vi "SngJntArmSim_GetCurrentDraw.vi"(11 "SingleJointArmSim":T1 {"GearBox"."Jr_KgM2" format="%13.5p"; "GearBox"."L_H" format="%13.5p"; "GearBox"."Kt_NMPerAmp" format="%13.5p"; "GearBox"."KvINV_RadPerSecPerVolt" format="%13.5p"; "GearBox"."R_Ohms" format="%13.5p"; "GearBox"."FreeSpeed_RadPerSec" format="%13.5p"; "GearBox"."FreeCurrent_Amps" format="%13.5p"; "GearBox"."StallCurrent_Amps" format="%13.5p"; "GearBox"."StallTorque_NM" format="%13.5p"; "GearBox"."nominalVoltage_Volts" format="%13.5p"}) -> (3 "Current_Amps":dbl)   [LabVIEW 2019, in "Trajectory_Library.lvlib"]
doc: "Returns the arm current draw.\n \nInputs:\n - SingleJointArmSim -- updated system data cluster\n\nOutputs:\n - Current_Amps -- The aram current draw. (Amps)"
uses:
  Trajectory_Library.lvlib
  SINGLE_JOINT_ARM_SIM.ctl
  LINEAR_SYSTEM_SIM.ctl
  LINEAR_SYSTEM.ctl
  <vilib>/Analysis/Matrix/Datatypes/RealMatrix.ctl
  DCMOTOR.CTL
  <vilib>/Analysis/Matrix/NI_Matrix.lvlib
panel:
  # "<States, 1>"
  # "<Outputs, 1>"
  # "<Inputs, 1>"
  # "<Outputs, 1>"
  # "<States,States>"
  # "<States,Inputs>"
  # "<Outputs,States>"
  # "<Outputs,Inputs>"
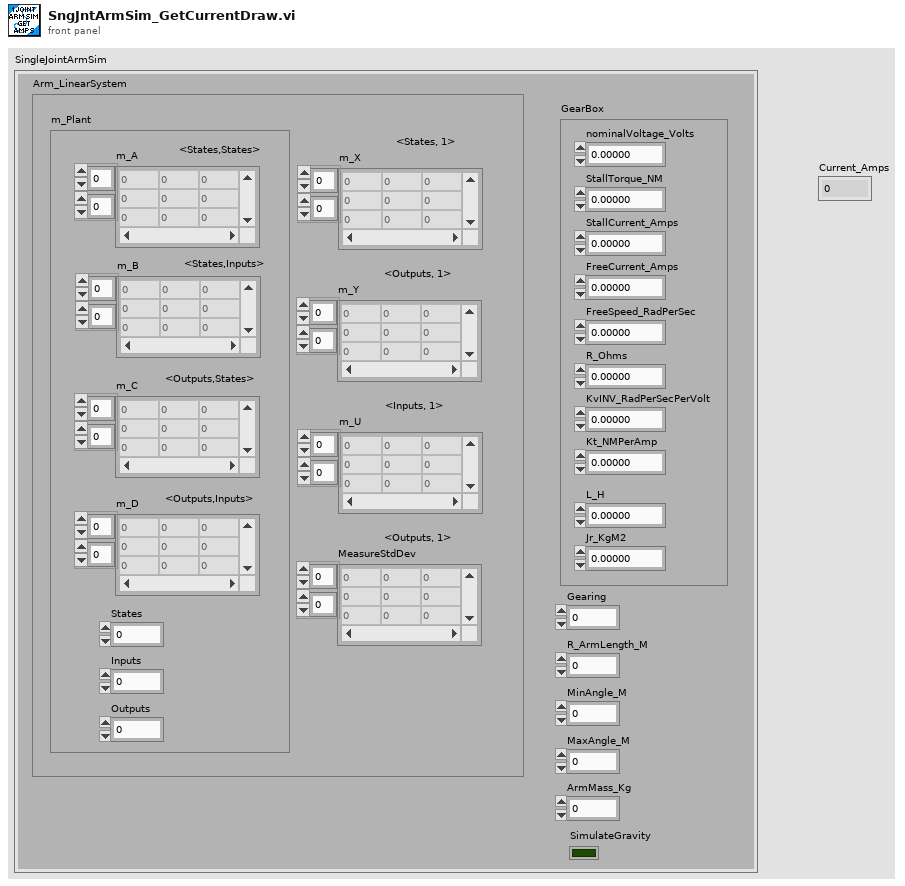
[diagram p1: front panel]
types:
  T1 = typedef "Trajectory_Library.lvlib/SINGLE_JOINT_ARM_SIM.ctl" = cluster{"Arm_LinearSystem":T2, "GearBox":T5, "Gearing":dbl, "R_ArmLength_M":dbl, "MinAngle_M":dbl, "MaxAngle_M":dbl, "ArmMass_Kg":dbl, "SimulateGravity":bool}
  T2 = typedef "Trajectory_Library.lvlib/LINEAR_SYSTEM_SIM.ctl" = cluster{"m_Plant":T3, "m_X":T4, "m_Y":T4, "m_U":T4, "MeasureStdDev":T4}
  T3 = typedef "Trajectory_Library.lvlib/LINEAR_SYSTEM.ctl" = cluster{"m_A":T4, "m_B":T4, "m_C":T4, "m_D":T4, "States":i32, "Inputs":i32, "Outputs":i32}
  T4 = typedef "NI_Matrix.lvlib/RealMatrix.ctl" = dbl[][]
  T5 = typedef "Trajectory_Library.lvlib/DCMOTOR.CTL" = cluster{"nominalVoltage_Volts":dbl, "StallTorque_NM":dbl, "StallCurrent_Amps":dbl, "FreeCurrent_Amps":dbl, "FreeSpeed_RadPerSec":dbl, "R_Ohms":dbl, "KvINV_RadPerSecPerVolt":dbl, "Kt_NMPerAmp":dbl, "L_H":dbl, "Jr_KgM2":dbl}
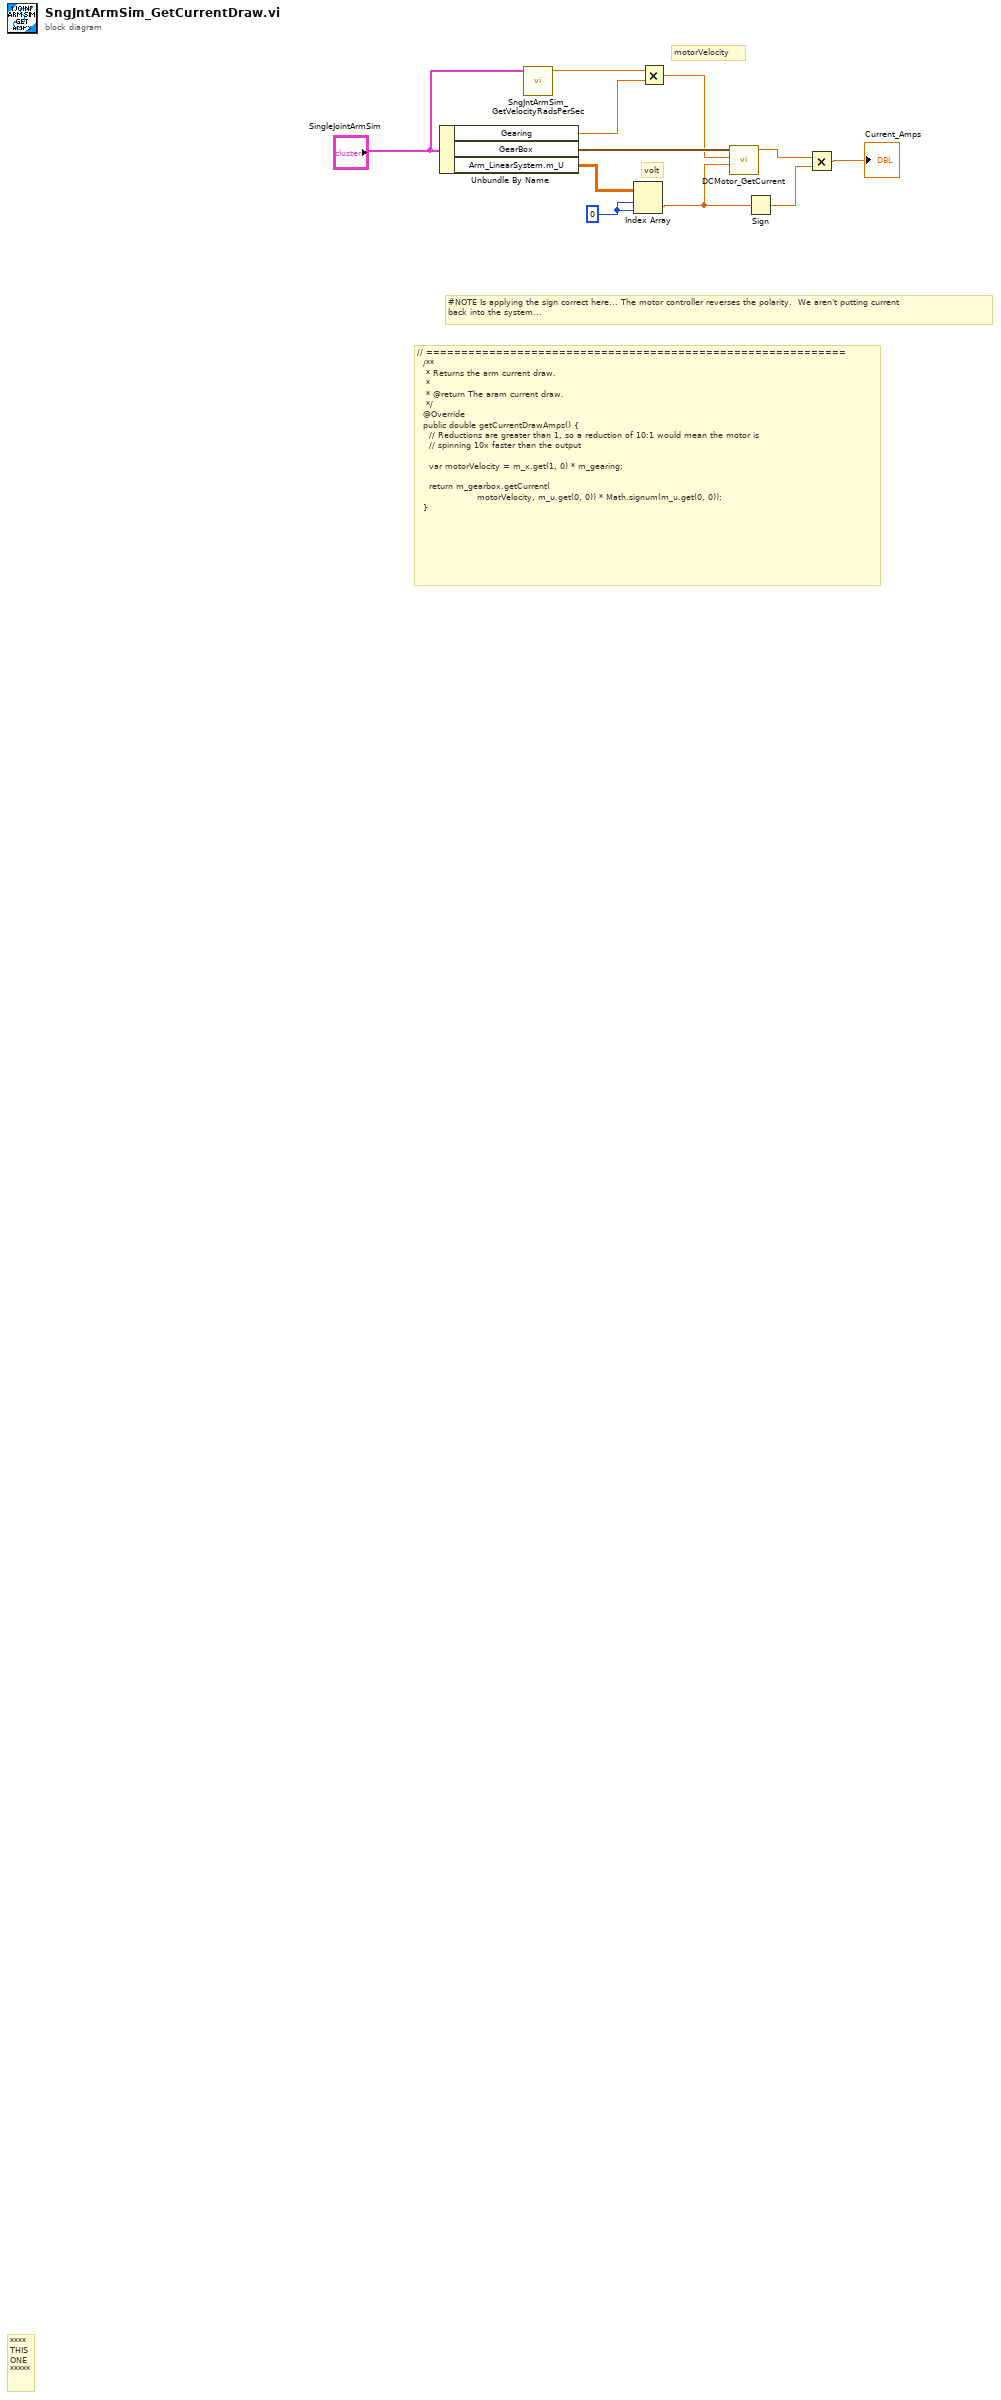
[diagram p0: block diagram]
diagram:
  w10 = 0 ("index (row)")
  # "motorVelocity"
  # "#NOTE Is applying the sign correct here... The motor controller reverses the polarity.  We aren't putting current\nback into the system..."
  # "volt"
  # "// ============================================================\n  /**\n   * Returns the arm current draw.\n   *\n   * @return The aram current draw.\n   */\n  @Override\n  public double getCurrentDrawAmps() {\n    // Reductions are greater than 1, so a reduction of 10:1 would mean the motor is\n    // spinning 10x faster than the output\n\n    var motorVelocity = m_x.get(1, 0) * m_gearing;\n\n    return m_gearbox.getCurrent(\n                    motorVelocity, m_u.get(0, 0)) * Math.signum(m_u.get(0, 0));\n  }"
  # "****\nTHIS\nONE\n*****"
  n1 = Unbundle By Name("SingleJointArmSim") -> ("Gearing"=w11:dbl, "GearBox"=w8:T5, "Arm_LinearSystem.m_U"=w9:T4)
  n2 = call "SngJntArmSim_GetVelocityRadsPerSec.vi"("singleJointArmSim"="SingleJointArmSim") -> ("Velocity_RadsPerSec"=w1:dbl)  [unwired: 10 in]
  n3 = Index Array(array=w9, index (row)=w10, index (col)=w10) -> (element=w6:dbl)
  n4 = Multiply(x=w1, y=w11) -> (x*y=w7:dbl)
  n5 = call "DCMotor_GetCurrent.vi"("VoltageInput_Volts"=w6, "Speed_RadPerSec"=w7, "DCMOTOR"=w8) -> ("Current_Amps"=w5:dbl)  [unwired: 8 in]
  n6 = Sign(1:w6) -> (0:w4:dbl)
  n7 = Multiply(x=w5, y=w4) -> (x*y=→"Current_Amps":dbl)
